vi "Fpga-U8-Array-U64.vi"(10 "data":u8[](array[numeric]), 11 "U8[] in":u8[](array[numeric])=[0, 0, 0, 0, 0, 0, 0, 0]) -> (3 "U64 out":u64)   [LabVIEW 2017]
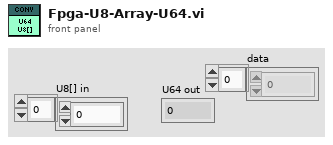
[diagram p1: front panel]
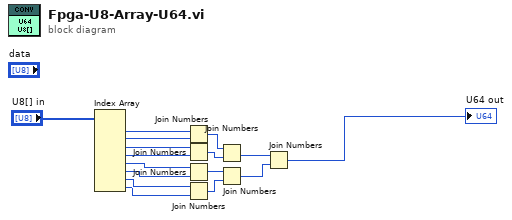
[diagram p0: block diagram]
diagram:
  n1 = Index Array(array="U8[] in") -> (element #1=w15:u8, element #2=w14:u8, element #3=w13:u8, element #4=w12:u8, element #5=w11:u8, element #6=w10:u8, element #7=w9:u8, element #8=w8:u8)  [unwired: 8 in]
  n2 = Join Numbers(hi=w15, lo=w14) -> ((hi.lo)=w4:u16)
  n3 = Join Numbers(hi=w13, lo=w12) -> ((hi.lo)=w5:u16)
  n4 = Join Numbers(hi=w11, lo=w10) -> ((hi.lo)=w6:u16)
  n5 = Join Numbers(hi=w9, lo=w8) -> ((hi.lo)=w7:u16)
  n6 = Join Numbers(hi=w4, lo=w5) -> ((hi.lo)=w2:u32)
  n7 = Join Numbers(hi=w6, lo=w7) -> ((hi.lo)=w3:u32)
  n8 = Join Numbers(hi=w2, lo=w3) -> ((hi.lo)=→"U64 out":u64)
